vi "Test_HelloWorld_Utf8Encoding.vi"() -> (0 "Array of Error Description":T1)   [LabVIEW 2019]
uses:
  gRPC_ATS/TestUtility/utility.llb/array of error description.ctl
  gRPC_ATS/TestUtility/utility.llb/error description.ctl
  gRPC_ATS/TestUtility/utility.llb/error type.ctl
  examples/helloworld/helloworld_client/RPC Messages/helloworld_HelloRequest.ctl
  690210b7-9fc1-4805-899f-f09b8e1640af.vi
  5de259ab-c1b1-450f-bfec-a70fb412634c.vi
  <vilib>/gRPC/LabVIEW gRPC Library/Server API/Translate Protobuf Error.vi
  <vilib>/AdvancedString/1D String Array to Delimited String.vi
  <vilib>/gRPC/LabVIEW gRPC Library/Server API/Server/Get Server DLL Path.vi
  examples/helloworld/helloworld_client/helloworld_client.lvlib
panel:
  out "Pass":bool
  in  "error in (no error)":errorcluster
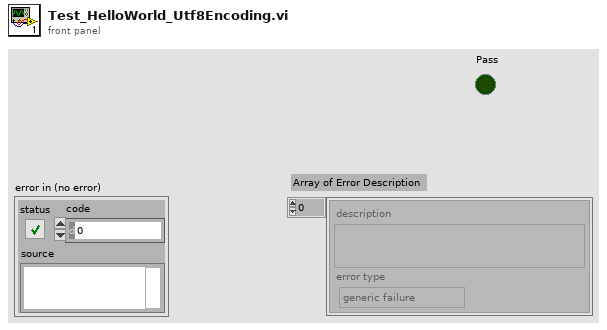
[diagram p1: front panel]
types:
  T1 = typedef "array of error description.ctl" = T2[]
  T2 = typedef "error description.ctl" = cluster{"description":string, "error type":T3}
  T3 = typedef "error type.ctl" = enum32{"generic failure", "boundary case", "precision", "expected error"}
  T4 = typedef "grpc-lvsupport-release.lvlib/grpcId.ctl" = u64
  T5 = typedef "helloworld_client.lvlib/helloworld_HelloRequest.ctl" = cluster{"name":string}
  T6 = typedef "grpc-lvsupport-release.lvlib/Any.ctl" = cluster{"Type Url":string, "Bytes":u8[]}
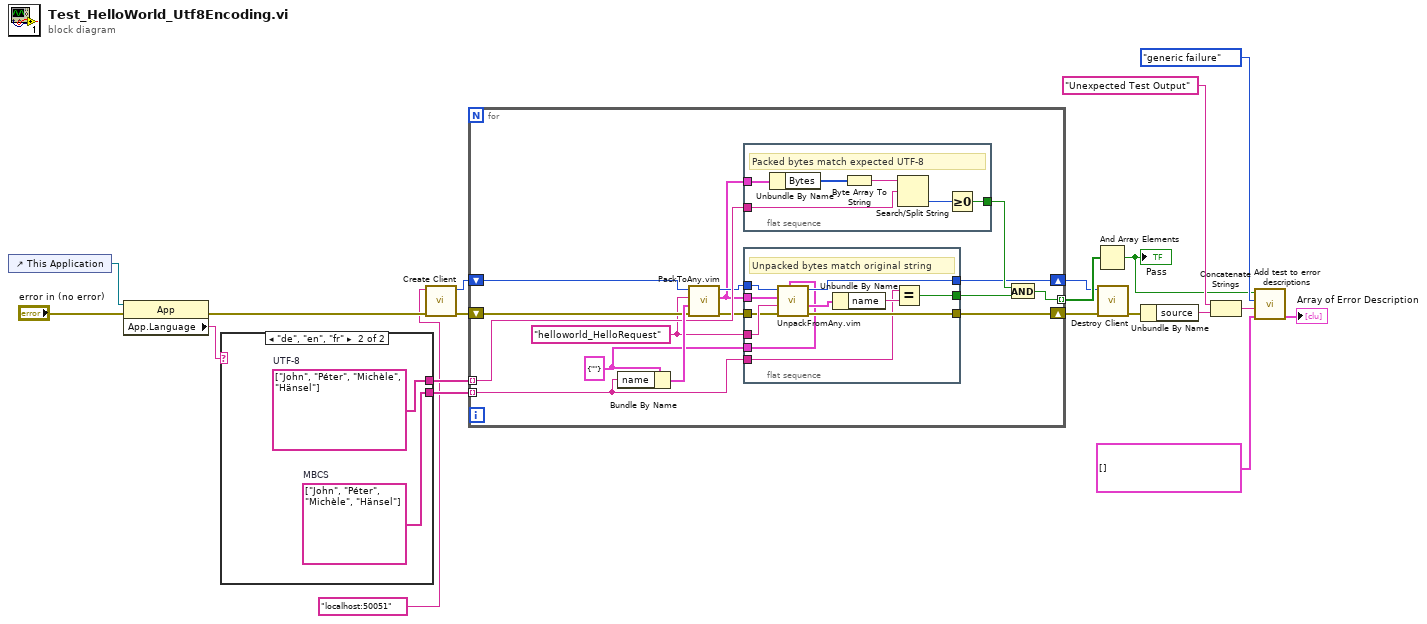
[diagram p0: block diagram]
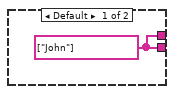
[diagram p2: hidden frame]
diagram:
  n1 = control-ref of="This Application"() -> (w12:refnum<vi>)
  n2 = property class="App"(reference=w12, error in="error in (no error)") -> (error out=w7:errorcluster, "App.Language"=w11:string)  [unwired: 1 out]
  n3 = case shown="\"de\", \"en\", \"fr\"" w11 {
    tunnel: [w21 w23] -> w10
    tunnel: [w21 w22] -> w9
    frame Default {
      w21 = string[] ["John"]
    }
    frame "de", "en", "fr" {
      w22 = string[] ["John", "Péter", "Michèle", "Hänsel"]  # UTF-8
      w23 = string[] ["John", "Péter", "Michèle", "Hänsel"]  # MBCS
    }
  }
  n4 = call "Create Client.vi"("error in"=w7, "address"="localhost:50051") -> ("error out"=w6:errorcluster, "gRPC ID Out"=w5:T4)  [unwired: 8 in]
  n5 = for {
    tunnel: [w26] -> w14 mode=indexing
    shift-right: [w28] -> w4
    shift-left: w6 -> [w35]
    tunnel: w10 -> [w24] mode=indexing
    tunnel: w9 -> [w37] mode=indexing
    shift-right: [w32] -> w3
    shift-left: w5 -> [w34]
    w31 = "helloworld_HelloRequest" ("Message Type")
    w27 = T5 {"name"=""} ("helloworld_HelloRequest")
    n6 = Bundle By Name(cluster=w27, "name"=w24) -> (w38:T5)
    n7 = call "PackToAny.vim"("error in"=w35, "Data To Pack"=w38, "Message Type"=w31, "gRPCid in"=w34) -> ("error out"=w29:errorcluster, "Any"=w30:T6, "gRPCid out"=w33:u64)  [unwired: 5 in]
    n8 = flat-sequence {
      tunnel: w37 -> [w53]
      tunnel: [w51] -> w36
      tunnel: w30 -> [w50]
      frame #0 {
        # "Packed bytes match expected UTF-8"
        n9 = Unbundle By Name(w50) -> ("Bytes"=w55:u8[])
        n10 = Byte Array To String(unsigned byte array=w55) -> (string=w54:string)
        n11 = Search/Split String(string=w54, search string/char (-)=w53) -> (offset of match=w52:i32)  [unwired: 1 in, 2 out]
        n12 = Greater Or Equal To 0?(x=w52) -> (x >= 0?=w51:bool)
      }
    }
    n13 = flat-sequence {
      tunnel: w33 -> [w49]
      tunnel: [w48] -> w32
      tunnel: w31 -> [w47]
      tunnel: w30 -> [w46]
      tunnel: w29 -> [w45]
      tunnel: [w44] -> w28
      tunnel: w27 -> [w42]
      tunnel: [w41] -> w25
      tunnel: w24 -> [w39]
      frame #0 {
        # "Unpacked bytes match original string"
        n14 = call "UnpackFromAny.vim"("Data Type"=w42, "error in"=w45, "Message Type"=w47, "Any"=w46, "gRPCid in"=w49) -> ("error out"=w44:errorcluster, "Unpacked Value"=w43:T5, "gRPCid out"=w48:u64)  [unwired: 4 in]
        n15 = Unbundle By Name(w43) -> ("name"=w40:string)
        n16 = Equal?(x=w39, y=w40) -> (x = y?=w41:bool)
      }
    }
    n17 = And(x=w36, y=w25) -> (x .and. y?=w26:bool)
  }
  n18 = And Array Elements(Boolean array=w14) -> (logical AND=w13:bool)
  "Pass" <- w13
  n19 = call "Destroy Client.vi"("error in"=w4, "gRPC ID"=w3) -> ("error out"=w2:errorcluster)  [unwired: 9 in]
  n20 = Unbundle By Name(w2) -> ("source"=w16:string)
  n21 = Concatenate Strings("Unexpected Test Output" ("string"), w16) -> (w17:string)
  n22 = call "Add test to error descriptions.vi"("error descriptions in"=T1 [], "error string"=w17, "error type"=error_type."generic failure", "pass"=w13) -> ("error description out"=→"Array of Error Description":T1)  [unwired: 3 in]
